vi "Build Poly Path - Serialize Data.vi"(1 "Directory":path) -> (0 "Path to Serialize ADAS Data.vi":path)   [LabVIEW 2020]
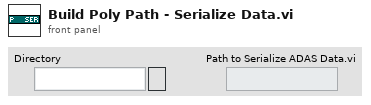
[diagram p1: front panel]
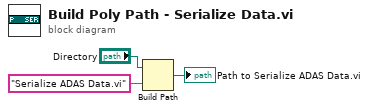
[diagram p0: block diagram]
diagram:
  n1 = Build Path(base path="Directory", name or relative path="Serialize ADAS Data.vi" ("Selector Name")) -> (appended path=→"Path to Serialize ADAS Data.vi":path)
